vi "Meas_ROI_Translated_From_Ellipse_Center.vi"(9 "ROI Descriptor":T1 {"Contours"."Type" items=["No Selection", "Point", "Line", "Rectangle", "Oval", "Polygon", "Freehand Region", "Annulus", "Unused2", "Unused3", "Broken Line", "Freehand Line", "Rotated Rectangle"]}, 10 "Straight Edges":T2(array[cluster]), 11 "Ellipse Center":cluster{"Center X":dbl, "Center Y":dbl}) -> (3 "Translated ROI":T3)   [LabVIEW 2019, in "Algorithm.lvclass"]
uses:
  FrameworkOverrides/Algorithm.lvclass
panel:
  out "Angle (Pixel)":dbl
types:
  T1 = typedef "ROI Descriptor" = cluster{"Global Rectangle":i32[], "Contours":cluster{"ID":enum32{"External", "Internal"}, "Type":u32, "Coordinates":i32[]}[]}
  T2 = cluster{"Point1 (Pixels)":cluster{"X":sgl, "Y":sgl}, "Point2 (Pixels)":cluster{"X":sgl, "Y":sgl}, "Point1 (Real-World)":cluster{"X":sgl, "Y":sgl}, "Point2 (Real-World)":cluster{"X":sgl, "Y":sgl}, "Angle (Pixel)":dbl, "Angle (Real-World)":dbl, "Score":dbl, "Straightness":dbl, "Average SNR (db)":dbl, "Calibration Valid":bool}[]
  T3 = cluster{"Left":dbl, "Top":dbl, "Right":dbl, "Bottom":dbl, "Angle":dbl}
  T4 = cluster{"ID":enum32{"External", "Internal"}, "Type":u32, "Coordinates":i32[]}[]
  T5 = cluster{"ID":enum32{"External", "Internal"}, "Type":u32, "Coordinates":i32[]}
  T6 = cluster{"Coordinates[0]":i32, "Coordinates[1]":i32, "Coordinates[2]":i32, "Coordinates[3]":i32, "Coordinates[4]":i32}
  T7 = cluster{"Point1 (Pixels)":cluster{"X":sgl, "Y":sgl}, "Point2 (Pixels)":cluster{"X":sgl, "Y":sgl}, "Point1 (Real-World)":cluster{"X":sgl, "Y":sgl}, "Point2 (Real-World)":cluster{"X":sgl, "Y":sgl}, "Angle (Pixel)":dbl, "Angle (Real-World)":dbl, "Score":dbl, "Straightness":dbl, "Average SNR (db)":dbl, "Calibration Valid":bool}
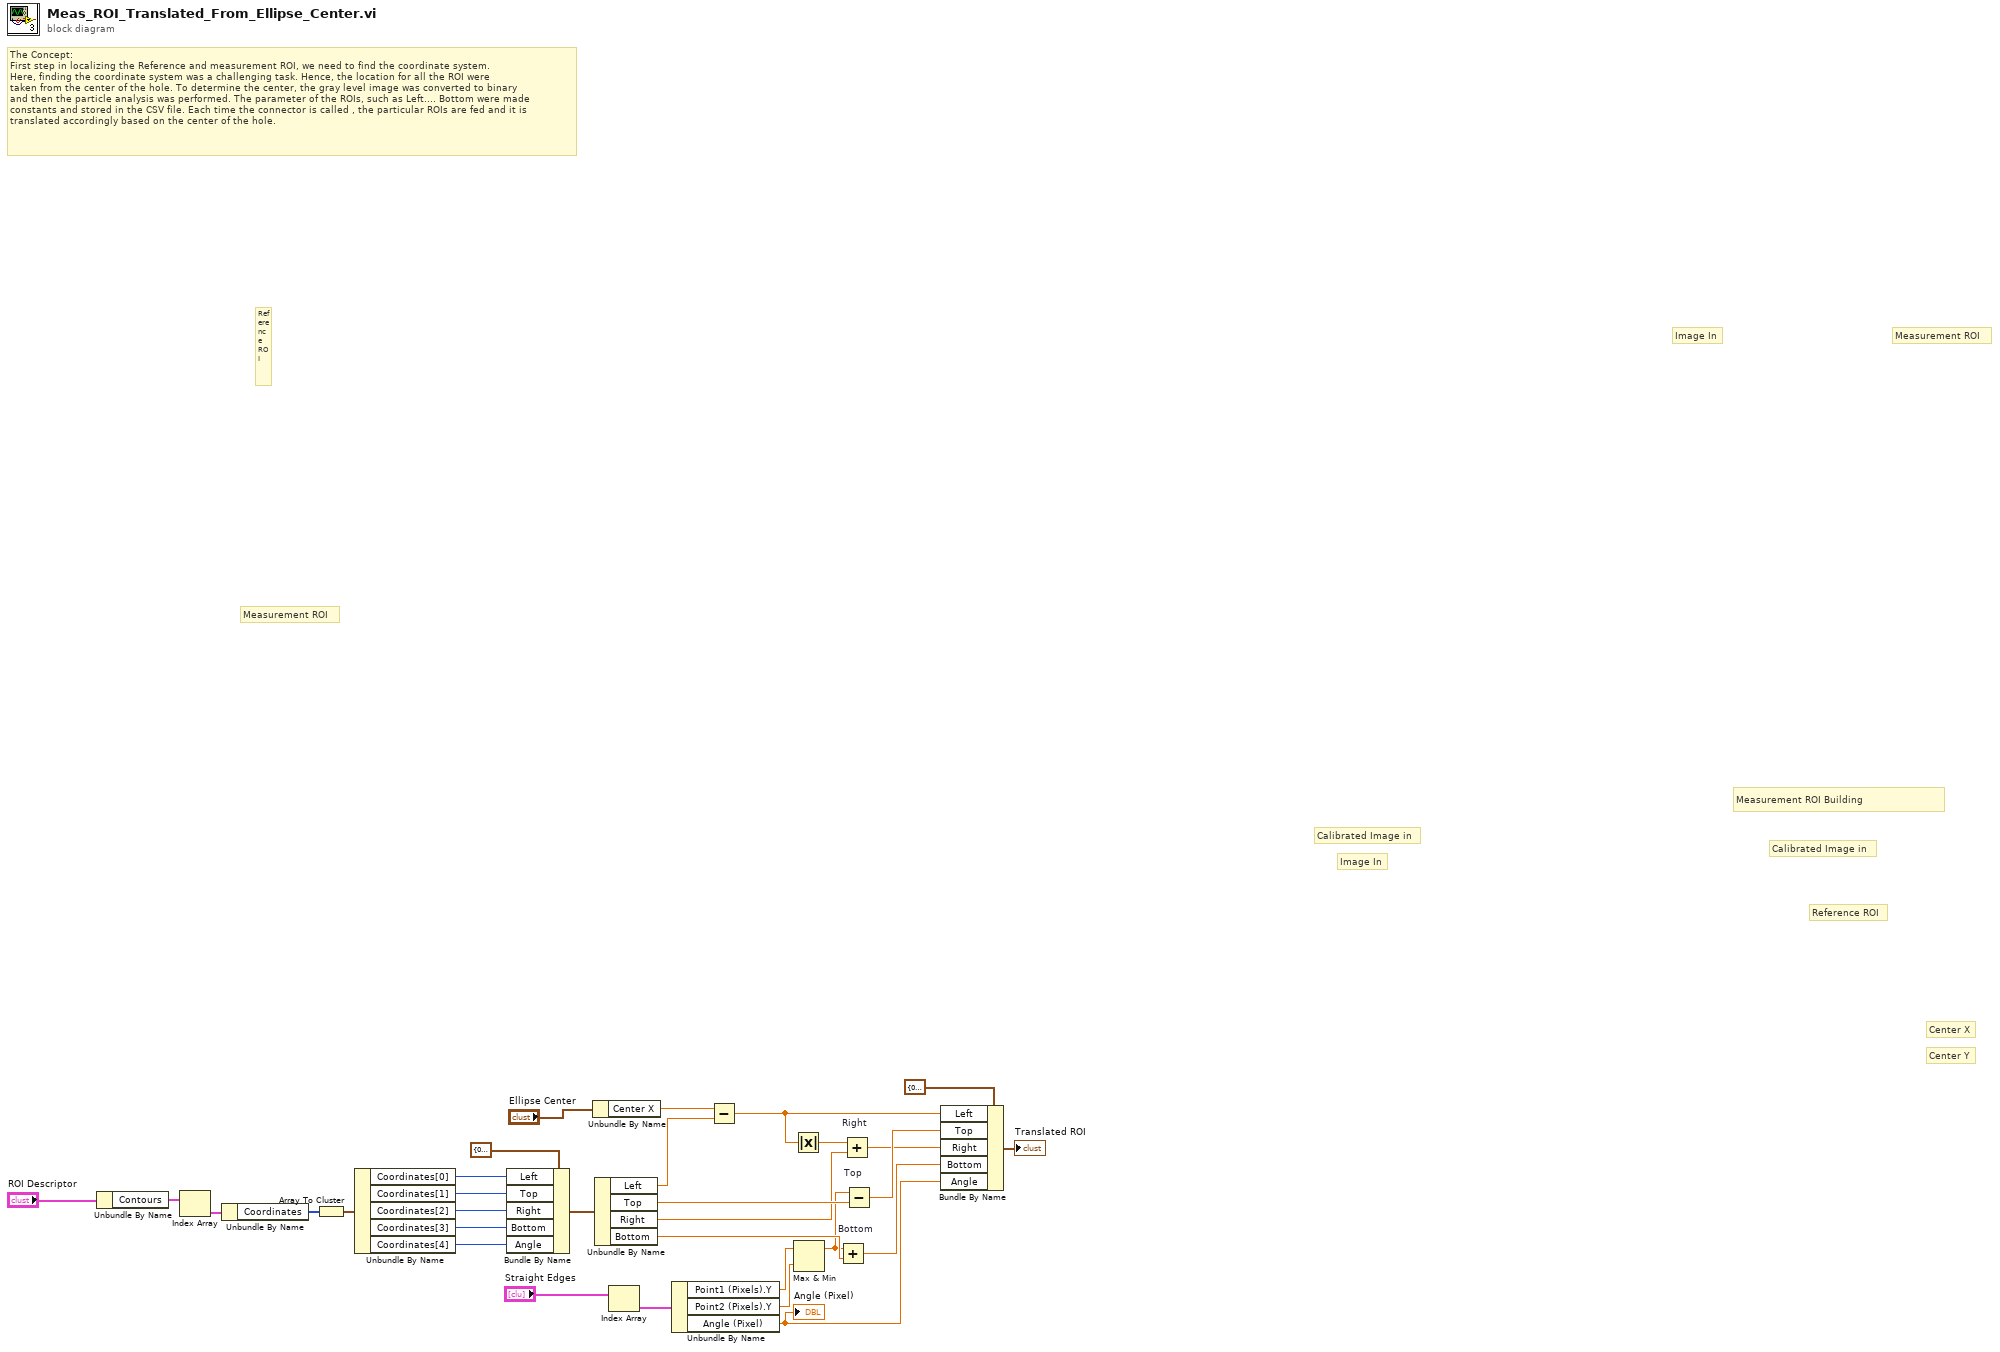
[diagram p0: block diagram]
diagram:
  # "The Concept:\nFirst step in localizing the Reference and measurement ROI, we need to find the coordinate system.\nHere, finding the coordinate system was a challenging task. Hence, the location for all the ROI were \ntaken from the center of the hole. To determine the center, the gray level image was converted to binary\nand then the particle analysis was performed. The parameter of the ROIs, such as Left.... Bottom were made \nconstants and stored in the CSV file. Each time the connector is called , the particular ROIs are fed and it is\ntranslated accordingly based on the center of the hole."
  # "Image In"
  # "Calibrated Image in"
  # "Image In"
  # "Calibrated Image in"
  # "Center Y"
  # "Center X"
  # "Reference ROI"
  # "Measurement ROI"
  # "Reference ROI"
  # "Measurement ROI"
  # "Measurement ROI Building"
  n1 = Unbundle By Name("ROI Descriptor") -> ("Contours"=w13:T4)
  n2 = Index Array(array=w13) -> (element=w14:T5)  [unwired: 1 in]
  n3 = Unbundle By Name(w14) -> ("Coordinates"=w15:i32[])
  n4 = Array To Cluster(array=w15) -> (cluster=w6:T6)
  n5 = Unbundle By Name "Unbundle By Name"(w6) -> ("Coordinates[0]"=w8:i32, "Coordinates[1]"=w9:i32, "Coordinates[2]"=w10:i32, "Coordinates[3]"=w11:i32, "Coordinates[4]"=w12:i32)
  n6 = Bundle By Name(cluster=T3 {"Left"=0.0, "Top"=0.0, "Right"=0.0, "Bottom"=0.0, "Angle"=0.0} ("Measurement ROI-1 Before transformation"), "Left"=w8, "Top"=w9, "Right"=w10, "Bottom"=w11, "Angle"=w12) -> (w5:T3)
  n7 = Unbundle By Name("Ellipse Center") -> ("Center X"=w19:dbl)
  n8 = Unbundle By Name(w5) -> ("Left"=w25:dbl, "Top"=w24:dbl, "Right"=w23:dbl, "Bottom"=w22:dbl)
  n9 = Index Array(array="Straight Edges") -> (element=w21:T7)  [unwired: 1 in]
  n10 = Unbundle By Name(w21) -> ("Point1 (Pixels).Y"=w18:sgl, "Point2 (Pixels).Y"=w17:sgl, "Angle (Pixel)"=w20:dbl)
  "Angle (Pixel)" <- w20
  n11 = Subtract(x=w19, y=w25) -> (x-y=w29:dbl)
  n12 = Absolute Value(x=w29) -> (abs(x)=w31:dbl)
  n13 = Max & Min(x=w18, y=w17) -> (max(x,y)=w16:sgl)  [unwired: 1 out]
  n14 = Add "Bottom"(x=w16, y=w22) -> (x+y=w26:dbl)
  n15 = Add "Right"(x=w31, y=w23) -> (x+y=w27:dbl)
  n16 = Subtract "Top"(x=w16, y=w24) -> (x-y=w28:dbl)
  n17 = Bundle By Name(cluster=T3 {"Left"=0.0, "Top"=0.0, "Right"=0.0, "Bottom"=0.0, "Angle"=0.0} ("input cluster"), "Left"=w29, "Top"=w28, "Right"=w27, "Bottom"=w26, "Angle"=w20) -> (→"Translated ROI":T3)
